vi "NewAutoBegin.vi"   [LabVIEW 2023]
uses:
  NewAutoGlobals.vi
types:
  T1 = typedef "NewAutoStepTypedef.ctl" = cluster{"Enum":T2, "Timeout":dbl, "Param1":dbl, "Param2":dbl, "Param3":dbl, "Function":string}
  T2 = typedef "NewAutoStepTypeEnum.ctl" = enum16{"DriveStraight", "DriveTurn", "FollowAbsoluteTrajectory", "FollowRelativeTrajectory", "AutoWait", "ElevToRest", "ElevToFloor", "ElevToSource", "ElevToL1", "ElevToL2", "ElevToL3", "ElevToL4", "ElevToAlgae1", "ElevToAlgae2", "ElevToBarge", "ElevCancel", "IntakeCoral", "IntakeAlgae", "IntakeDepositCoral", "IntakeDepositAlgae", "IntakeCancel", "ElevRestWait", "ElevFloorWait", "ElevSourceWait", "ElevL1Wait", "ElevL2Wait", "ElevAlgae1Wait", "ElevL3Wait", "ElevAlgae2Wait", "ElevL4Wait", "ElevBargeWait", "IntakeWait", "FollowAbsTrajWithTimedCmd", "FollowRelTrajWithTimedCmd"}
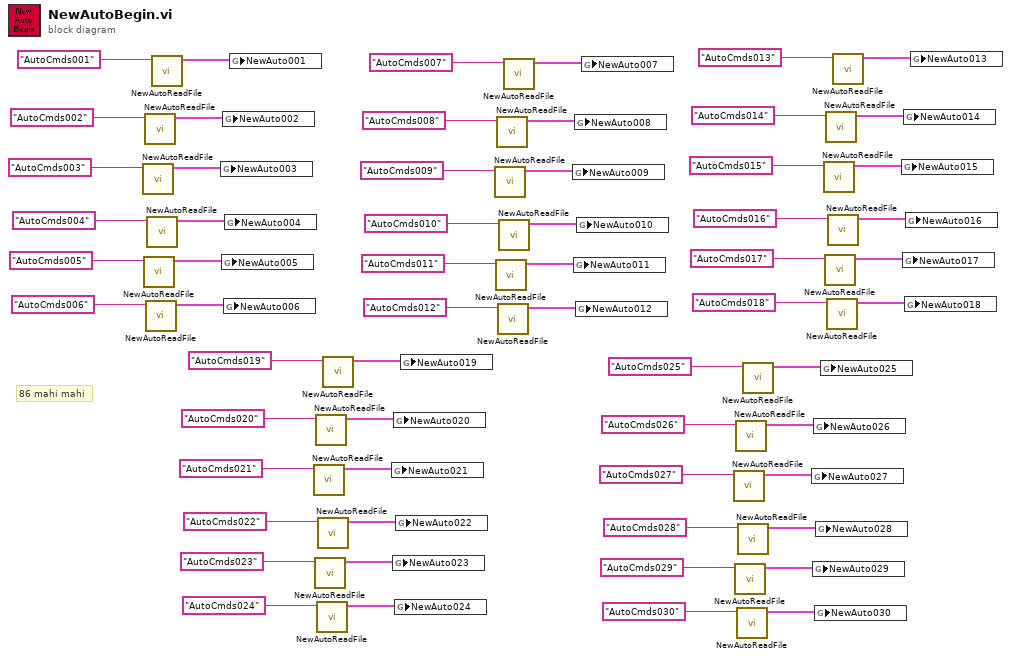
[diagram p0: block diagram]
diagram:
  # "86 mahi mahi"
  n1 = call "NewAutoReadFile.vi"("FileName"="AutoCmds003") -> ("outTRAJECTORY"=w56:T1[])  [unwired: 8 in, 2 out]
  n2 = call "NewAutoReadFile.vi"("FileName"="AutoCmds005") -> ("outTRAJECTORY"=w52:T1[])  [unwired: 8 in, 2 out]
  n3 = call "NewAutoReadFile.vi"("FileName"="AutoCmds002") -> ("outTRAJECTORY"=w58:T1[])  [unwired: 8 in, 2 out]
  n4 = call "NewAutoReadFile.vi"("FileName"="AutoCmds006") -> ("outTRAJECTORY"=w50:T1[])  [unwired: 8 in, 2 out]
  n5 = call "NewAutoReadFile.vi"("FileName"="AutoCmds004") -> ("outTRAJECTORY"=w54:T1[])  [unwired: 8 in, 2 out]
  n6 = call "NewAutoReadFile.vi"("FileName"="AutoCmds001") -> ("outTRAJECTORY"=w60:T1[])  [unwired: 8 in, 2 out]
  n7 = global write "NewAutoGlobals.vi" "NewAuto003"(w56) -> ()
  n8 = global write "NewAutoGlobals.vi" "NewAuto005"(w52) -> ()
  n9 = global write "NewAutoGlobals.vi" "NewAuto002"(w58) -> ()
  n10 = global write "NewAutoGlobals.vi" "NewAuto006"(w50) -> ()
  n11 = global write "NewAutoGlobals.vi" "NewAuto004"(w54) -> ()
  n12 = global write "NewAutoGlobals.vi" "NewAuto001"(w60) -> ()
  n13 = call "NewAutoReadFile.vi"("FileName"="AutoCmds021") -> ("outTRAJECTORY"=w20:T1[])  [unwired: 8 in, 2 out]
  n14 = call "NewAutoReadFile.vi"("FileName"="AutoCmds023") -> ("outTRAJECTORY"=w16:T1[])  [unwired: 8 in, 2 out]
  n15 = call "NewAutoReadFile.vi"("FileName"="AutoCmds020") -> ("outTRAJECTORY"=w22:T1[])  [unwired: 8 in, 2 out]
  n16 = call "NewAutoReadFile.vi"("FileName"="AutoCmds024") -> ("outTRAJECTORY"=w14:T1[])  [unwired: 8 in, 2 out]
  n17 = call "NewAutoReadFile.vi"("FileName"="AutoCmds022") -> ("outTRAJECTORY"=w18:T1[])  [unwired: 8 in, 2 out]
  n18 = call "NewAutoReadFile.vi"("FileName"="AutoCmds019") -> ("outTRAJECTORY"=w24:T1[])  [unwired: 8 in, 2 out]
  n19 = global write "NewAutoGlobals.vi" "NewAuto021"(w20) -> ()
  n20 = global write "NewAutoGlobals.vi" "NewAuto023"(w16) -> ()
  n21 = global write "NewAutoGlobals.vi" "NewAuto020"(w22) -> ()
  n22 = global write "NewAutoGlobals.vi" "NewAuto024"(w14) -> ()
  n23 = global write "NewAutoGlobals.vi" "NewAuto022"(w18) -> ()
  n24 = global write "NewAutoGlobals.vi" "NewAuto019"(w24) -> ()
  n25 = call "NewAutoReadFile.vi"("FileName"="AutoCmds009") -> ("outTRAJECTORY"=w44:T1[])  [unwired: 8 in, 2 out]
  n26 = call "NewAutoReadFile.vi"("FileName"="AutoCmds011") -> ("outTRAJECTORY"=w40:T1[])  [unwired: 8 in, 2 out]
  n27 = call "NewAutoReadFile.vi"("FileName"="AutoCmds008") -> ("outTRAJECTORY"=w46:T1[])  [unwired: 8 in, 2 out]
  n28 = call "NewAutoReadFile.vi"("FileName"="AutoCmds012") -> ("outTRAJECTORY"=w38:T1[])  [unwired: 8 in, 2 out]
  n29 = call "NewAutoReadFile.vi"("FileName"="AutoCmds010") -> ("outTRAJECTORY"=w42:T1[])  [unwired: 8 in, 2 out]
  n30 = call "NewAutoReadFile.vi"("FileName"="AutoCmds007") -> ("outTRAJECTORY"=w48:T1[])  [unwired: 8 in, 2 out]
  n31 = global write "NewAutoGlobals.vi" "NewAuto009"(w44) -> ()
  n32 = global write "NewAutoGlobals.vi" "NewAuto011"(w40) -> ()
  n33 = global write "NewAutoGlobals.vi" "NewAuto008"(w46) -> ()
  n34 = global write "NewAutoGlobals.vi" "NewAuto012"(w38) -> ()
  n35 = global write "NewAutoGlobals.vi" "NewAuto010"(w42) -> ()
  n36 = global write "NewAutoGlobals.vi" "NewAuto007"(w48) -> ()
  n37 = call "NewAutoReadFile.vi"("FileName"="AutoCmds027") -> ("outTRAJECTORY"=w8:T1[])  [unwired: 8 in, 2 out]
  n38 = call "NewAutoReadFile.vi"("FileName"="AutoCmds029") -> ("outTRAJECTORY"=w4:T1[])  [unwired: 8 in, 2 out]
  n39 = call "NewAutoReadFile.vi"("FileName"="AutoCmds026") -> ("outTRAJECTORY"=w10:T1[])  [unwired: 8 in, 2 out]
  n40 = call "NewAutoReadFile.vi"("FileName"="AutoCmds030") -> ("outTRAJECTORY"=w2:T1[])  [unwired: 8 in, 2 out]
  n41 = call "NewAutoReadFile.vi"("FileName"="AutoCmds028") -> ("outTRAJECTORY"=w6:T1[])  [unwired: 8 in, 2 out]
  n42 = call "NewAutoReadFile.vi"("FileName"="AutoCmds025") -> ("outTRAJECTORY"=w12:T1[])  [unwired: 8 in, 2 out]
  n43 = global write "NewAutoGlobals.vi" "NewAuto027"(w8) -> ()
  n44 = global write "NewAutoGlobals.vi" "NewAuto029"(w4) -> ()
  n45 = global write "NewAutoGlobals.vi" "NewAuto026"(w10) -> ()
  n46 = global write "NewAutoGlobals.vi" "NewAuto030"(w2) -> ()
  n47 = global write "NewAutoGlobals.vi" "NewAuto028"(w6) -> ()
  n48 = global write "NewAutoGlobals.vi" "NewAuto025"(w12) -> ()
  n49 = call "NewAutoReadFile.vi"("FileName"="AutoCmds015") -> ("outTRAJECTORY"=w32:T1[])  [unwired: 8 in, 2 out]
  n50 = call "NewAutoReadFile.vi"("FileName"="AutoCmds017") -> ("outTRAJECTORY"=w28:T1[])  [unwired: 8 in, 2 out]
  n51 = call "NewAutoReadFile.vi"("FileName"="AutoCmds014") -> ("outTRAJECTORY"=w34:T1[])  [unwired: 8 in, 2 out]
  n52 = call "NewAutoReadFile.vi"("FileName"="AutoCmds018") -> ("outTRAJECTORY"=w26:T1[])  [unwired: 8 in, 2 out]
  n53 = call "NewAutoReadFile.vi"("FileName"="AutoCmds016") -> ("outTRAJECTORY"=w30:T1[])  [unwired: 8 in, 2 out]
  n54 = call "NewAutoReadFile.vi"("FileName"="AutoCmds013") -> ("outTRAJECTORY"=w36:T1[])  [unwired: 8 in, 2 out]
  n55 = global write "NewAutoGlobals.vi" "NewAuto015"(w32) -> ()
  n56 = global write "NewAutoGlobals.vi" "NewAuto017"(w28) -> ()
  n57 = global write "NewAutoGlobals.vi" "NewAuto014"(w34) -> ()
  n58 = global write "NewAutoGlobals.vi" "NewAuto018"(w26) -> ()
  n59 = global write "NewAutoGlobals.vi" "NewAuto016"(w30) -> ()
  n60 = global write "NewAutoGlobals.vi" "NewAuto013"(w36) -> ()
